vi "_Rohde & Schwarz VNA Tree.vi"   [LabVIEW 2011]
uses:
  VNA Command.ctl
panel:
  # "See Diagram"
types:
  T1 = typedef "VNA Command.ctl" = enum16{"LOAD", "INITIALIZE", "PRESET", "GET STIMULUS", "SET STIMULUS", "GET CALIBRATION", "CALIBRATE", "RESTORE", "MEASURE", "RELEASE", "UNLOAD", "CONFIRM", "SORT"}
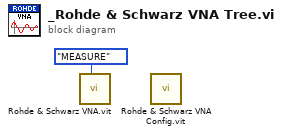
[diagram p0: block diagram]
diagram:
  n1 = call "Rohde & Schwarz VNA.vit"("VNA Command"=VNA_Command."MEASURE") -> ()  [unwired: 5 in, 6 out]
  n2 = call "Rohde & Schwarz VNA Config.vit"() -> ()  [unwired: 2 in, 10 out]
